vi "Snapshot Images.vi"(8 "error in (no error)":errorcluster) -> (0 "error IO":errorcluster, 3 "Saved Path":path)   [LabVIEW 2020]
uses:
  Global Variables/gl_Images.vi
  <vilib>/vision/NI_Vision_Development_Module.lvlib
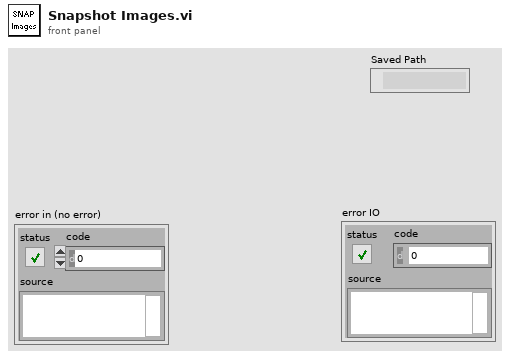
[diagram p1: front panel]
types:
  T1 = typedef "Image Type" = u32
  T2 = typedef "IMAQ Image.ctl" = refnum<image>
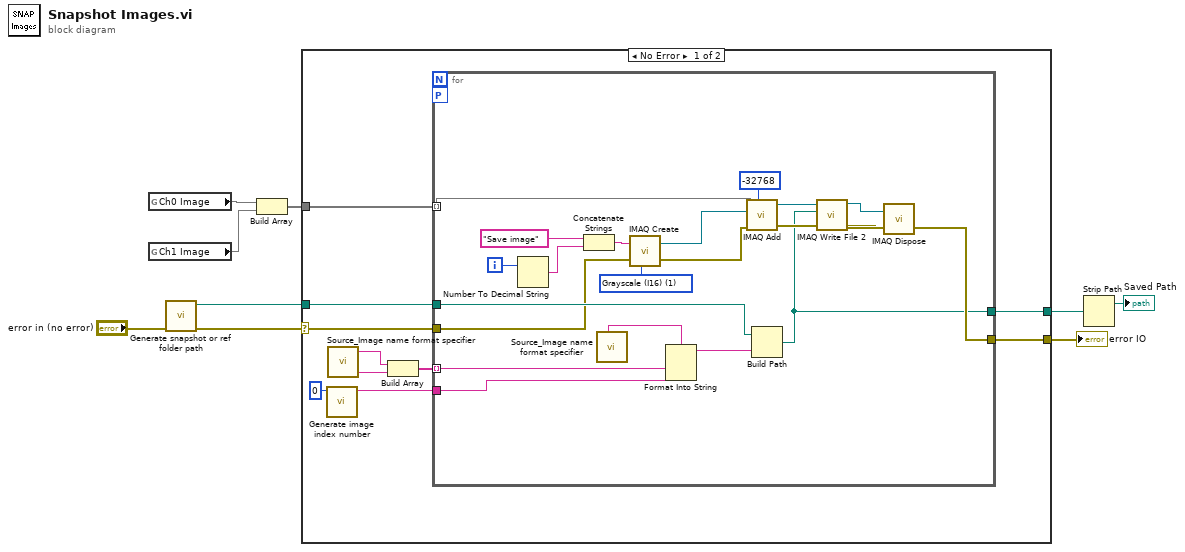
[diagram p0: block diagram]
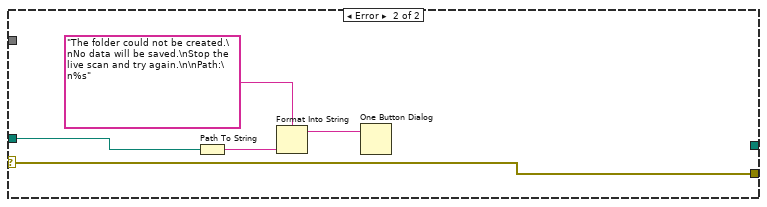
[diagram p2: hidden frame]
diagram:
  n1 = global read "gl_Images.vi" "Ch0 Image"() -> (w5)
  n2 = global read "gl_Images.vi" "Ch1 Image"() -> (w4)
  n3 = call "Generate snapshot or ref folder path.vi"("error in (no error)"="error in (no error)") -> ("error out"=w7:errorcluster, "Snapshot folder path"=w6:path)  [unwired: 9 in]
  n4 = Build Array(w5, w4) -> (w3:void[])
  n5 = case shown="No Error" w7 {
    selector: w7 -> [w18 w41]
    tunnel: w6 -> [w19 w45]
    tunnel: [w17 w41] -> w9
    tunnel: w3 -> [w16 _]
    tunnel: [w10 _] -> w2
    frame No Error {
      n6 = call "Generate image index number.vi"("FOR loop iteration or existing number of files"=0) -> ("Number in string representation (padded with zeroes)"=w12:string)  [unwired: 10 in]
      n7 = call "Source_Image name format specifier.vi"() -> ("Red channel name"=w14:string, "Green channel name"=w13:string)  [unwired: 5 in, 1 out]
      n8 = Build Array(w14, w13) -> (w15:string[])
      n9 = for {
        tunnel: w19 -> [w32]
        tunnel: w18 -> [w30]
        tunnel: w16 -> [w40] mode=indexing
        tunnel: w15 -> [w28] mode=indexing
        tunnel: [w39] -> w17
        workers-P: _ -> [_]
        tunnel: w12 -> [w26]
        tunnel: [w20] -> w10
        i -> [w33]
        w38 = T1 1 items=["Grayscale (U8)", "Grayscale (I16)", "Grayscale (SGL)", "Complex (CSG)", "RGB (U32)", "HSL (U32)", "RGB (U64)"] ("Image Type")
        n10 = Number To Decimal String(number=w33) -> (decimal integer string=w36:string)  [unwired: 1 in]
        n11 = Concatenate Strings("Save image" ("Image Name"), w36) -> (w35:string)
        n12 = call "Source_Image name format specifier.vi"() -> ("Z-Stack Image name format specifier"=w27:string)  [unwired: 5 in, 2 out]
        n13 = call "IMAQ Create"("Image Name"=w35, "Image Type"=w38, "error in (no error)"=w30) -> ("New Image"=w34:T2, "error out"=w31:errorcluster)  [unwired: 2 in]
        n14 = Format Into String(format string=w27, w28, w26) -> (resulting string=w29:string)  [unwired: 2 in, 1 out]
        n15 = call "IMAQ Add"("Image Src A"=w40, "Constant"=i16 -32768, "Image Dst"=w34, "error in (no error)"=w31) -> ("Image Dst Out"=w24:T2, "error out"=w21:errorcluster)  [unwired: 3 in]
        n16 = Build Path(base path=w32, name or relative path=w29) -> (appended path=w20:path)
        n17 = call-poly "IMAQ Write File 2"("error in (no error)"=w21, "File Path"=w20, "Image"=w24) -> ("error out"=w22:errorcluster, "Image Out (duplicate)"=w23:T2)  [unwired: 7 in]
        n18 = call "IMAQ Dispose"("Image"=w23, "error in (no error)"=w22) -> ("error out"=w39:errorcluster)  [unwired: 4 in]
      }
    }
    frame Error {
      n19 = Path To String(path=w45) -> (string=w43:string)
      n20 = Format Into String(format string="The folder could not be created.\nNo data will be saved.\nStop the live scan and try again.\n\nPath:\n%s", w43) -> (resulting string=w42:string)  [unwired: 2 in, 1 out]
      n21 = One Button Dialog(message=w42) -> ()  [unwired: 1 in, 1 out]
    }
  }
  "error IO" <- w9
  n22 = Strip Path(path=w2) -> (stripped path=→"Saved Path":path)  [unwired: 1 out]
